vi "S2C_FPGA_Global.vi"() -> ()   [LabVIEW 2015]
panel:
  out "C1/P3/B1":bool
  out "C1/P3/B0":bool
  out "C1/P2/B5":bool
  out "C1/P2/B4":bool
  out "C1/P2/B1":bool
  out "C1/P2/B0":bool
  out "C1/P1/B7":bool
  out "C1/P1/B6":bool
  out "C1/P1/B5":bool
  out "C1/P1/B4":bool
  out "C1/P1/B3":bool
  out "C1/P1/B2":bool
  out "C1/P1/B1":bool
  out "C1/P1/B0":bool
  out "C1/P0/B7":bool
  out "C1/P0/B6":bool
  out "C1/P0/B5":bool
  out "C1/P0/B4":bool
  out "C1/P0/B3":bool
  out "C1/P0/B2":bool
  out "C1/P0/B1":bool
  out "C1/P0/B0":bool
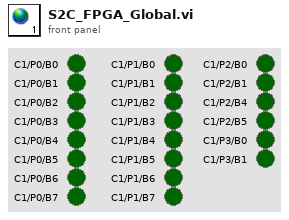
[diagram p1: front panel]
diagram:
